vi "Set dll parameter.vi"(7 "Parameter Cluster":T1, 8 "error in (no error)":errorcluster, 11 "path in":path) -> (0 "error out":errorcluster, 2 "phaserange in Pi":i32=16, 3 "path out":path)   [LabVIEW 2023]
uses:
  dllparameter.ctl
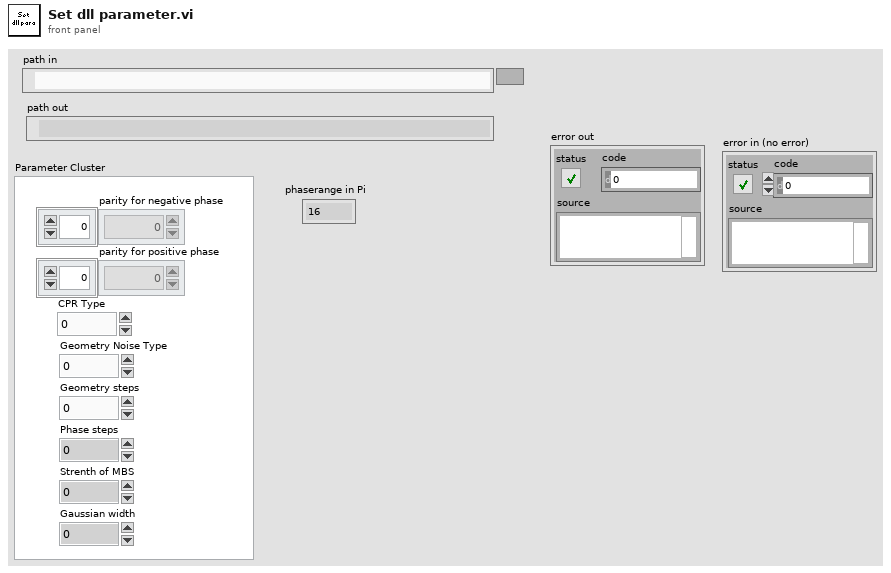
[diagram p1: front panel]
types:
  T1 = typedef "dllparameter.ctl" = cluster{"Gaussian width":dbl, "Strenth of MBS":dbl, "Phase steps":i32, "Geometry steps":i32, "Geometry Noise Type":u16, "CPR Type":dbl, "parity for positive phase":dbl[], "parity for negative phase ":dbl[]}
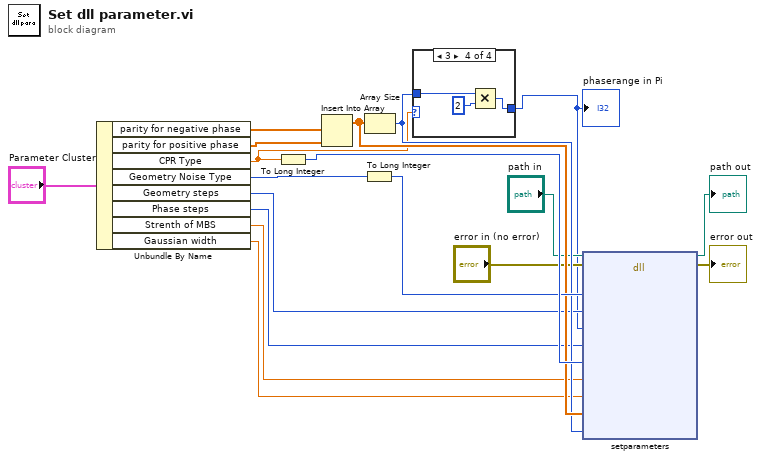
[diagram p0: block diagram]
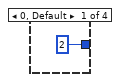
[diagram p2: hidden frame]
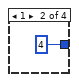
[diagram p3: hidden frame]
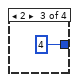
[diagram p4: hidden frame]
diagram:
  n1 = Unbundle By Name("Parameter Cluster") -> ("parity for negative phase"=w12:dbl[], "parity for positive phase"=w11:dbl[], "CPR Type"=w10:dbl, "Geometry Noise Type"=w9:u16, "Geometry steps"=w8:i32, "Phase steps"=w7:i32, "Strenth of MBS"=w6:dbl, "Gaussian width"=w5:dbl)
  n2 = To Long Integer(number=w10) -> (32bit integer=w18:i32)
  n3 = Insert Into Array(array=w12, new element=w11) -> (w16:dbl[])  [unwired: 1 in]
  n4 = To Long Integer(number=w9) -> (32bit integer=w17:i32)
  n5 = Array Size(array=w16) -> (size(s)=w15:i32)
  n6 = case shown="3" w10 {
    tunnel: [2 4 4 w22] -> w1
    tunnel: w15 -> [_ _ _ w24]
    frame 0, Default {
    }
    frame 1 {
    }
    frame 2 {
    }
    frame 3 {
      n7 = Multiply(x=w24, y=2) -> (x*y=w22:i32)
    }
  }
  "phaserange in Pi" <- w1
  n8 = dll-call lib="C:/Users/yg/Box/Guang Yue uiuc research box folder/computation/S-TI-S jj simulation c/Release/ygDLL.dll" fn="setparameters"(path in="path in", error in="error in (no error)", "Jnt"=w17, "Nw"=w8, "PhaseRange"=w1, "nphase"=w7, "cpr"=w18, "a"=w6, "gw"=w5, "parity"=w16, "parity_l"=w15) -> (path out=→"path out":path, error out=→"error out":errorcluster)  [unwired: 11 in]
